vi "ABB make Report browse.vi"(2 "result string":string, 3 "WebBrowser":refnum<k7>(container), 4 "report template folder":path) -> (0 "Report  path":path, 1 "report out":T1)   [LabVIEW 2017]
uses:
  <vilib>/Utility/NIReport.llb/Generate Report Object Reference.ctl
  <vilib>/Utility/NIReport.llb/NI_report.lvclass
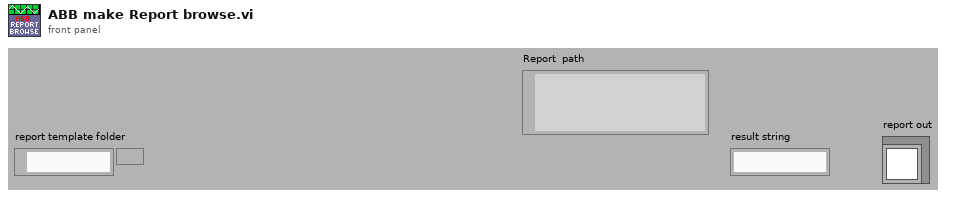
[diagram p1: front panel]
types:
  T1 = typedef "Generate Report Object Reference.ctl" = refnum<class "NI_report.lvclass">
  T2 = cluster{"charset (-1)":i16, "weight (-1)":i16, "name":string, "size":string}
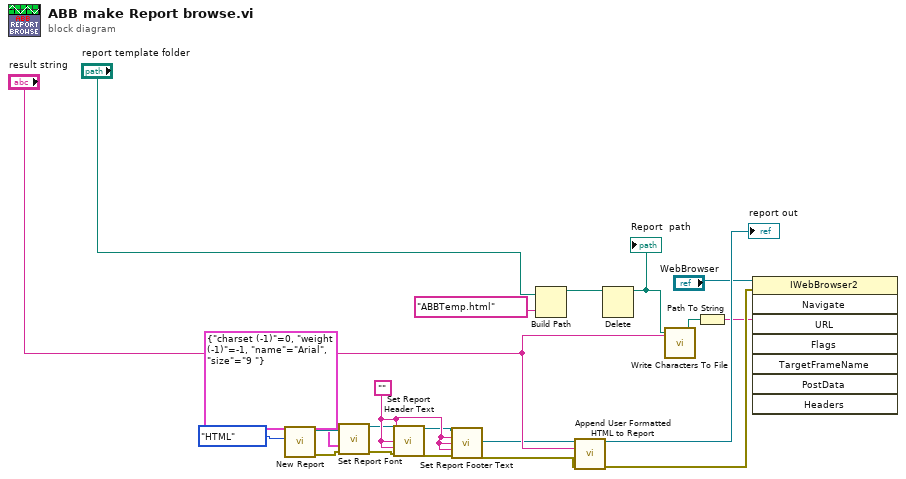
[diagram p0: block diagram]
diagram:
  w19 = ""
  n1 = call <vilib>:"New Report.vi"("report type"=enum16{"Standard Report", "HTML"}."HTML") -> ("report out"=w5:refnum<class "NI_report.lvclass">, "error out"=w4:errorcluster)  [unwired: 13 in]
  n2 = call-dynamic "Set Report Font.vi"("report in"=w5, "font settings"=T2 {"charset (-1)"=0, "weight (-1)"=-1, "name"="Arial", "size"="9 "}, "error in (no error)"=w4) -> ("report out"=w3:refnum<class "NI_report.lvclass">, "error out"=w2:errorcluster)  [unwired: 10 in, 1 out]
  n3 = call-dynamic "Set Report Header Text.vi"("report in"=w3, "left header text"=w19, "center header text"=w19, "right header text"=w19, "error in (no error)"=w2) -> ("report out"=w15:refnum<class "NI_report.lvclass">, "error out"=w16:errorcluster)  [unwired: 9 in]
  n4 = call-dynamic "Set Report Footer Text.vi"("report in"=w15, "left footer text"=w19, "center footer text"=w19, "right footer text"=w19, "error in (no error)"=w16) -> ("report out"=w18:refnum<class "NI_report.lvclass">, "error out"=w17:errorcluster)  [unwired: 9 in]
  n5 = Build Path(base path="report template folder", name or relative path="ABBTemp.html") -> (appended path=w11:path)
  n6 = call-dynamic "Append User Formatted HTML to Report.vi"("report in"=w18, "HTML text"="result string", "error in (no error)"=w17) -> ("report out"=→"report out":refnum<class "NI_report.lvclass">, "error out"=w14:errorcluster)  [unwired: 11 in]
  n7 = Delete(path (use dialog)=w11) -> (deleted path=w12:path)  [unwired: 4 in, 2 out]
  "Report  path" <- w12
  n8 = call <vilib>:"Write Characters To File.vi"("character string"="result string", "file path (dialog if empty)"=w12) -> ("new file path (Not A Path if cancelled)"=w8:path)  [unwired: 3 in]
  n9 = Path To String(path=w8) -> (string=w9:string)
  n10 = invoke class="IWebBrowser2" method="Navigate"(reference="WebBrowser", error in=w14, "URL"=w9) -> ()  [unwired: 5 in, 8 out]
